vi "Hitrap_DiagnosticBoxGUI.status color.vi"(2 "Status":i32) -> (16 "Color":u32(colorbox))   [LabVIEW 2014, in "Hitrap_DiagnosticBoxGUI.lvlib"]
doc: "sets the color of status indicator.\n\nThis VI is used in the VI \"set color\""
uses:
  Hitrap_DiagnosticBoxGUI.lvlib
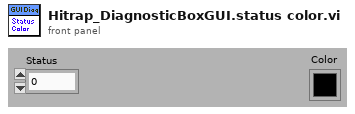
[diagram p1: front panel]
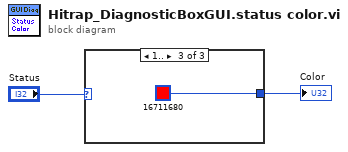
[diagram p0: block diagram]
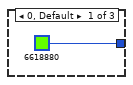
[diagram p2: hidden frame]
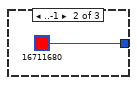
[diagram p3: hidden frame]
diagram:
  n1 = case shown="1.." "Status" {
    tunnel: [u32 6618880 u32 16711680 u32 16711680] -> w1
    frame 0, Default {
    }
    frame ..-1 {
    }
    frame 1.. {
    }
  }
  "Color" <- w1
